vi "Append Test.vi"(8 "error in":errorcluster, 11 "TDMS in":refnum<class "TDMS.lvclass">) -> (0 "error out":errorcluster, 3 "TDMS out":refnum<class "TDMS.lvclass">)   [LabVIEW 2019, in "TDMS.lvlib" / "TDMS.lvclass"]
uses:
  TDMS.lvclass
  TDMS.lvclass/TDMS.ctl
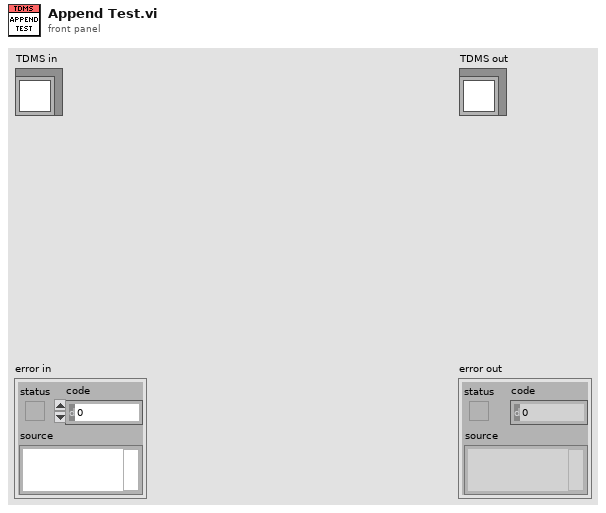
[diagram p1: front panel]
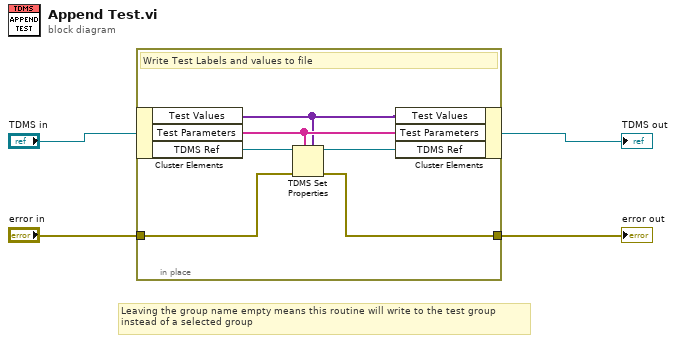
[diagram p0: block diagram]
diagram:
  # "Leaving the group name empty means this routine will write to the test group\ninstead of a selected group"
  n1 = in-place {
    in-place-border: [w10] -> w2
    in-place-border: "error in" -> [w9]
    # "Write Test Labels and values to file"
    n2 = in-place-cluster #1("TDMS in") -> ("Test Values"=w6:variant[], "Test Parameters"=w7:string[], "TDMS Ref"=w8:refnum<k34>)
    n3 = TDMS Set Properties(5:w6, 7:w7, 8:w9, 11:w8) -> (0:w10:errorcluster, 3:w5:refnum<k34>)  [unwired: 2 in, 2 out]
    n4 = in-place-cluster #1("Test Values"=w6, "Test Parameters"=w7, "TDMS Ref"=w5) -> (→"TDMS out":refnum<class "TDMS.lvclass">)
  }
  "error out" <- w2
